vi "0-10Vdc.vi"(8 "error in (no error)":errorcluster, 10 "Reg Array":u16[](array[numeric]), 11 "object in":refnum<class "Pressure-Transducer.lvclass">) -> (0 "error out":errorcluster, 1 "Array Size":i32, 2 "0-10Vdc Data":dbl[](array[numeric]), 3 "object out":refnum<class "Pressure-Transducer.lvclass">)   [LabVIEW 2021, in "Pressure-Transducer.lvclass"]
doc: "converts 0 to 10Vdc from modbus reg"
uses:
  Pressure-Transducer.lvclass
panel:
  # "Converts the Adam 4017 Reg\nto 0 to 10Vdc\nNo scaling"
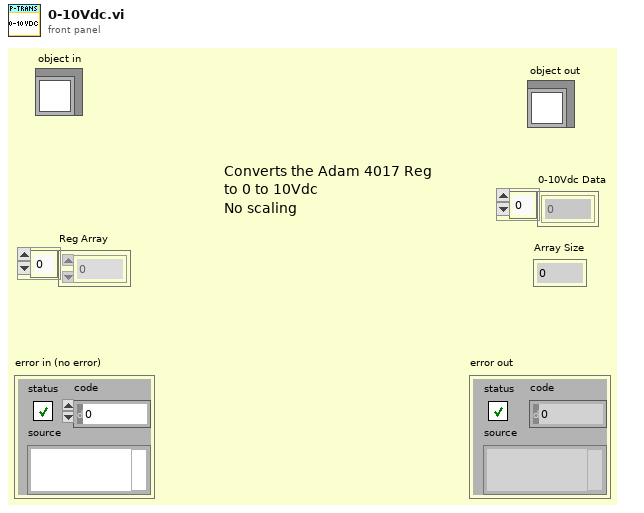
[diagram p1: front panel]
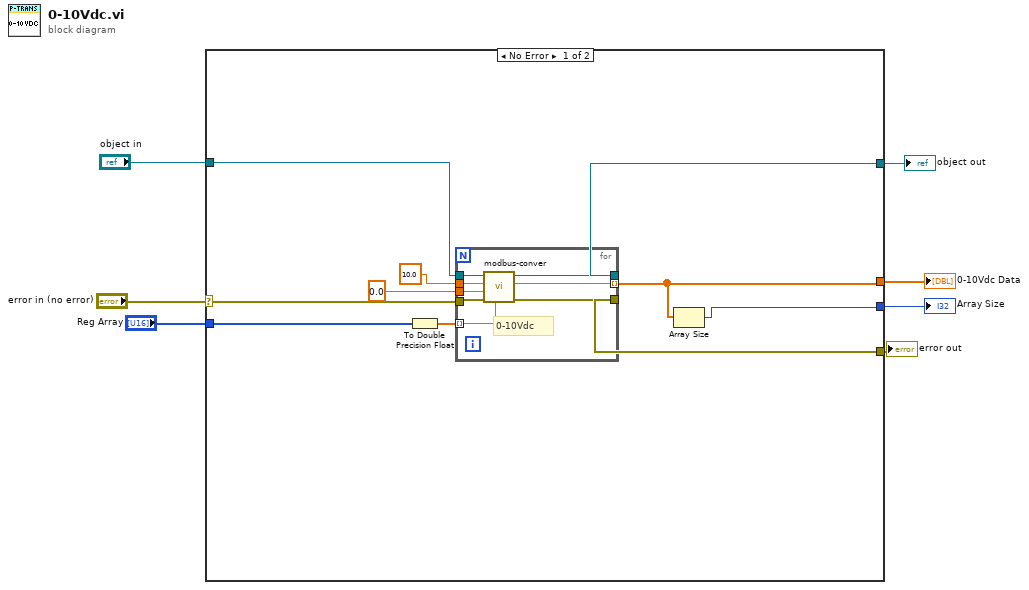
[diagram p0: block diagram]
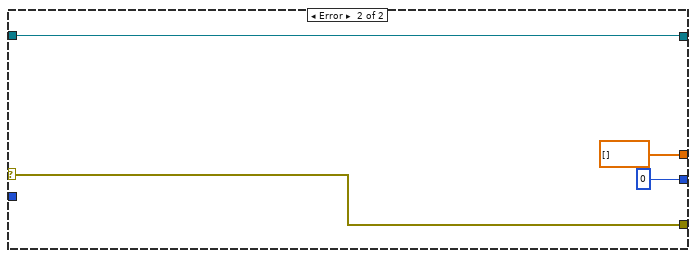
[diagram p2: hidden frame]
diagram:
  n1 = case shown="No Error" "error in (no error)" {
    selector: "error in (no error)" -> [w14 w29]
    tunnel: [w13 w29] -> w6
    tunnel: [w10 w28] -> w4
    tunnel: "object in" -> [w11 w28]
    tunnel: "Reg Array" -> [w12 _]
    tunnel: [w9 dbl[] []] -> w2
    tunnel: [w8 0] -> w1
    frame No Error {
      n2 = To Double Precision Float(number=w12) -> (double precision float=w17:dbl[])
      n3 = for {
        tunnel: w11 -> [w21]
        tunnel: 10.0 ("Scale Max Range") -> [w24]
        tunnel: 0.0 ("Scale Min range") -> [w23]
        tunnel: w14 -> [w25]
        tunnel: [w18] -> w9 mode=indexing
        tunnel: w17 -> [w22] mode=indexing
        tunnel: [w20] -> w10
        tunnel: [w19] -> w13
        # "0-10Vdc"
        n4 = call-dynamic "modbus-conver.vi"("Reg"=w22, "error in (no error)"=w25, "Scale Min range"=w23, "Scale Max Range"=w24, "object in"=w21) -> ("error out"=w19:errorcluster, "output"=w18:dbl, "object out"=w20:refnum<class "Pressure-Transducer.lvclass">)  [unwired: 4 in]
      }
      n5 = Array Size(array=w9) -> (size(s)=w8:i32)
    }
    frame Error {
    }
  }
  "error out" <- w6
  "object out" <- w4
  "0-10Vdc Data" <- w2
  "Array Size" <- w1
